vi "globals.vi"() -> ()   [LabVIEW 2013]
uses:
  qwtblvlib/TD Calculation Settings.ctl
  qwtblvlib/TD Uncertainty Calculation Method.ctl
  qwtblvlib/TD Correlation Calculation Settings.ctl
  qwtblvlib/TD DOF Calculation Settings.ctl
  qwtblvlib/TD MCM Calculation Settings.ctl
  qwtblvlib/TD MCM Calculation Method.ctl
  TD GUI Settings.ctl
  qwtblvlib/TD Backend Engine.ctl
  qwtblvlib/TD Algorithm Information.ctl
  qwtblvlib/TD Algorithm Information Input.ctl
  qwtblvlib/TD Algorithm Information Output.ctl
  qwtblvlib/QWTBLVLib.lvlib
panel:
  in  "settings cluster template":T12={"Calculation Settings"={"Strict"=FALSE, "Verbose"=TRUE, "Uncertainty Calculation Method"=enum."none", "Correlations"={"Required"=FALSE, "Generate"=FALSE}, "Degrees of Freedom"={"Required"=FALSE, "Generate"=FALSE}, "MCM Calculation Settings"={"Repeats"=100, "Verbose"=TRUE, "Parallelization method"=enum."Single Core", "Processors"=1, "Temporary directory"=".", "Randomize"=TRUE}}, "GUI Settings"={"Backend engine"=enum."Matlab by Script node", "QWTB Folder Path"=path ""}, "Data In"=[], "Available Algorithms"=[], "Current Algorithm"={"ID"="", "Name"="", "Description"="", "Citation"="", "Remarks"="", "License"="", "Inputs"=[], "Outputs"=[], "Provides GUF"=FALSE, "Provides MCM"=FALSE, "Full path"=""}, "Data Out"=[]} {"Calculation Settings"."MCM Calculation Settings"."Processors" min=0 step=1; "Calculation Settings"."MCM Calculation Settings"."Repeats" min=1 step=1}
  in  "settings filename":string="settings.xml"
  out "new data signal reference":refnum<vi>
  in  "Current Algorithm":T9
  in  "Data Out":T13(array[cluster])
  in  "Data In":T13(array[cluster])
  out "Available Algorithms":T9[](array[typedef])
  in  "GUI Settings":T7={"Backend engine"=enum."Matlab by Script node", "QWTB Folder Path"=path ""}
  in  "Calculation Settings":T1={"Strict"=FALSE, "Verbose"=TRUE, "Uncertainty Calculation Method"=enum."none", "Correlations"={"Required"=FALSE, "Generate"=FALSE}, "Degrees of Freedom"={"Required"=FALSE, "Generate"=FALSE}, "MCM Calculation Settings"={"Repeats"=100, "Verbose"=TRUE, "Parallelization method"=enum."Single Core", "Processors"=0, "Temporary directory"=".", "Randomize"=TRUE}} {"MCM Calculation Settings"."Processors" min=0 step=1; "MCM Calculation Settings"."Repeats" min=1 step=1}
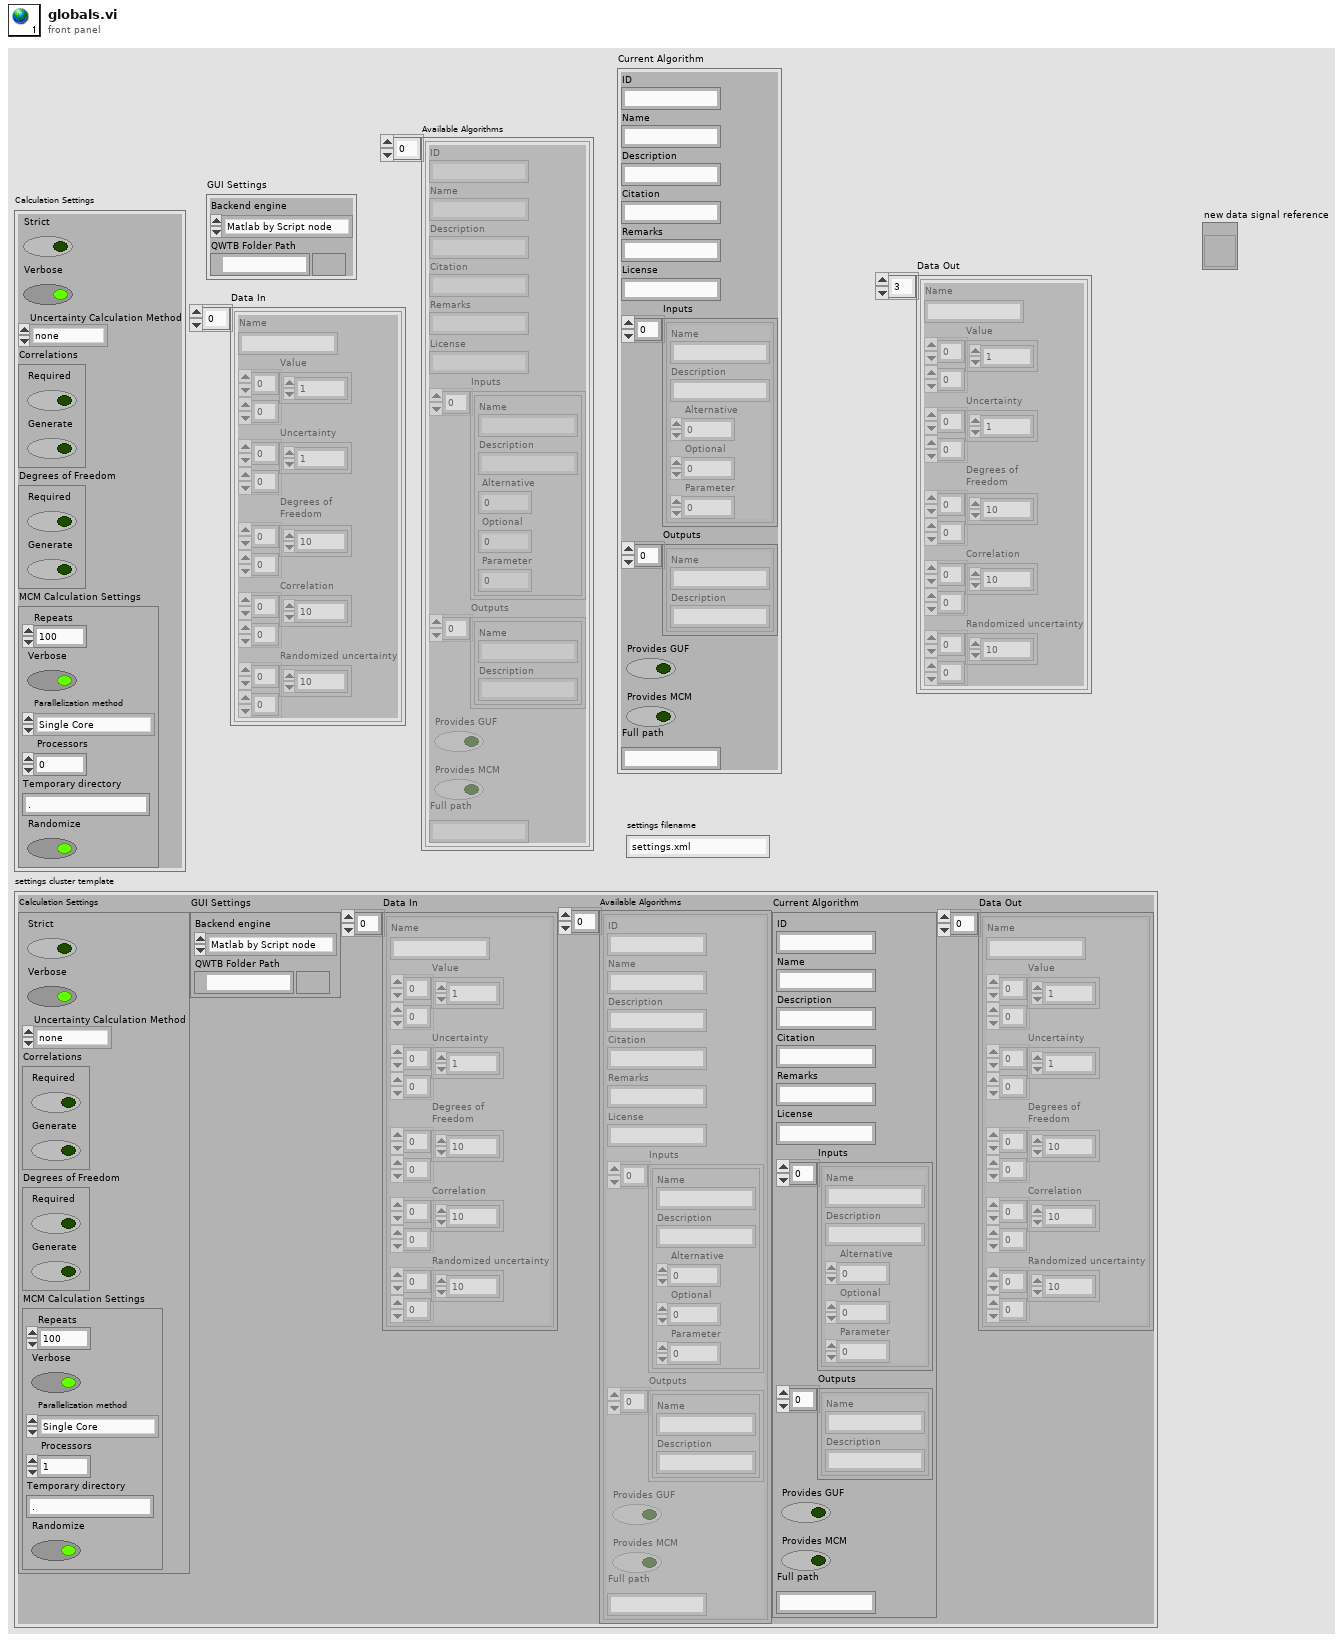
[diagram p1: front panel]
types:
  T1 = typedef "QWTBLVLib.lvlib/TD Calculation Settings.ctl" = cluster{"Strict":bool, "Verbose":bool, "Uncertainty Calculation Method":T2, "Correlations":T3, "Degrees of Freedom":T4, "MCM Calculation Settings":T5}
  T2 = typedef "QWTBLVLib.lvlib/TD Uncertainty Calculation Method.ctl" = enum16{"none", "GUF", "MCM"}
  T3 = typedef "QWTBLVLib.lvlib/TD Correlation Calculation Settings.ctl" = cluster{"Required":bool, "Generate":bool}
  T4 = typedef "QWTBLVLib.lvlib/TD DOF Calculation Settings.ctl" = cluster{"Required":bool, "Generate":bool}
  T5 = typedef "QWTBLVLib.lvlib/TD MCM Calculation Settings.ctl" = cluster{"Repeats":i32, "Verbose":bool, "Parallelization method":T6, "Processors":i32, "Temporary directory":string, "Randomize":bool}
  T6 = typedef "QWTBLVLib.lvlib/TD MCM Calculation Method.ctl" = enum16{"Single Core", "Multi Core", "Multi Station"}
  T7 = typedef "TD GUI Settings.ctl" = cluster{"Backend engine":T8, "QWTB Folder Path":path}
  T8 = typedef "QWTBLVLib.lvlib/TD Backend Engine.ctl" = enum16{"Matlab by Script node", "GNU Octave by GOLPI"}
  T9 = typedef "QWTBLVLib.lvlib/TD Algorithm Information.ctl" = cluster{"ID":string, "Name":string, "Description":string, "Citation":string, "Remarks":string, "License":string, "Inputs":T10[], "Outputs":T11[], "Provides GUF":bool, "Provides MCM":bool, "Full path":string}
  T10 = typedef "QWTBLVLib.lvlib/TD Algorithm Information Input.ctl" = cluster{"Name":string, "Description":string, "Alternative":i32, "Optional":i32, "Parameter":i32}
  T11 = typedef "QWTBLVLib.lvlib/TD Algorithm Information Output.ctl" = cluster{"Name":string, "Description":string}
  T12 = cluster{"Calculation Settings":T1, "GUI Settings":T7, "Data In":cluster{"Name":string, "Value":dbl[][], "Uncertainty":dbl[][], "Degrees of\nFreedom":dbl[][], "Correlation":dbl[][], "Randomized uncertainty":dbl[][]}[], "Available Algorithms":T9[], "Current Algorithm":T9, "Data Out":cluster{"Name":string, "Value":dbl[][], "Uncertainty":dbl[][], "Degrees of\nFreedom":dbl[][], "Correlation":dbl[][], "Randomized uncertainty":dbl[][]}[]}
  T13 = cluster{"Name":string, "Value":dbl[][], "Uncertainty":dbl[][], "Degrees of\nFreedom":dbl[][], "Correlation":dbl[][], "Randomized uncertainty":dbl[][]}[]
diagram:
